vi "Compile Save Data (SubVI).vi"(0 "Dispense Mode":T5(ring), 1 "Mass Chart":T4, 2 "Relay Control":T2, 3 "Dispense Setpoint (%)":dbl=2.5, 4 "Values":T6 {"Drain Time (s)" format="%.2f"; "Drain Rate (g/sec)" format="%.2f"; "Spray Mass Loss (g)" format="%.2f"; "Time Elapsed (s)" format="%.2f"; "Time Target (s)" format="%.2f"; "Dynamic Setpoint (g)" format="%.2f"; "Static Setpoint (g)" format="%.2f"; "Grams to Setpoint" format="%.2f"; "Adjusted Mass (g)" format="%.2f"; "Dispense Rate (g/sec)" format="%.2f"; "Fill Mass (g)" format="%.2f"; "Fill Rate (g/sec)" format="%.2f"}, 5 "Settings":T1={"ON Settings"={"Enable Dynamic Setpoint?"=TRUE, "Enable Dynamic Dispense Time?"=TRUE, "Enable Drain Rate Functions"=TRUE, "Dispense Sample Time (s)"=0.1, "Mass Average Samples"=20, "ON Timeout (sec)"=300.0, "1st Setpoint (% of Target)"=90.0, "2nd Setpoint (% of Target)"=95.0, "3rd Setpoint (% of Target)"=100.0, "Measure Dispense Delay (sec)"=10.0, "Minimum Spray Time (s)"=2.0, "Pump Reverse Time (s)"=10.0}, "OFF Settings"={"Drain Sample Time (s)"=0.1, "Drain Rate Ave Size"=100, "Drain Rate Limits (± g/sec)"=100.0, "Level Slope Range (± g/sec)"=0.05, "OFF Timeout (sec)"=300.0, "Near SP Slope Level (± g/sec)"=0.005, "Near Setpoint Threshold (%)"=99.0}, "Overshoot Settings"={"Time Limit (s)"=30.0, "Container MAX (g)"=1500.0, "Max FILL Slope (+/- g/sec)"=100.0, "% Overshot to Enable (>)"=3.0}, "FILL Timeout (s)"=300.0, "Full \nSettle Time (s)"=30.0, "Pre-Hydrate \nSpray Time (s)"=0.0, "Pre-Hydrate \nWait Time (s)"=10.0, "m Value "=1.0, "b Value"=0.0, "Enable Overshoot Adjust?"=FALSE} {"ON Settings"."Pump Reverse Time (s)" min=0.0 max=60.0; "OFF Settings"."Near SP Slope Level (± g/sec)" format="%.3g"; "OFF Settings"."Level Slope Range (± g/sec)" format="%.3g"}, 7 "Hydration (g)":dbl, 9 "Product Mass (g)":dbl, 11 "Product Values":T3) -> (14 "Data Array Output":string[](array[string]), 15 "Column Header Text Array":string[](array[string])=["Grams (SCB)", "Fill Target", "Dispense Target", "Relay (All)", "Relay1 (Spray)", "Relay2 (Fill)", "Relay3 (Drain)", "Relay4", "Relay5", "Relay6", "Relay7", "Dispense Mode", "Dispense Setpoint (%)", "Spray Timeout (s)", "Wait Timeout (s)", "Adjusted Mass (grams)", "Time Target (s)", "Dispense Rate (g/sec)", "Dynamic Setpoint (g)", "Measure Dispense Delay (s)", "Fill Mass (grams)", "Fill Rate (g/sec)", "Time Elapsed (s)", "Spray Mass Loss (g)"])   [LabVIEW 2011]
panel:
  # "ONLY ADJUST\nBOLD VALUES!"
  # "Corrected Mass = SDC Mass * m + b"
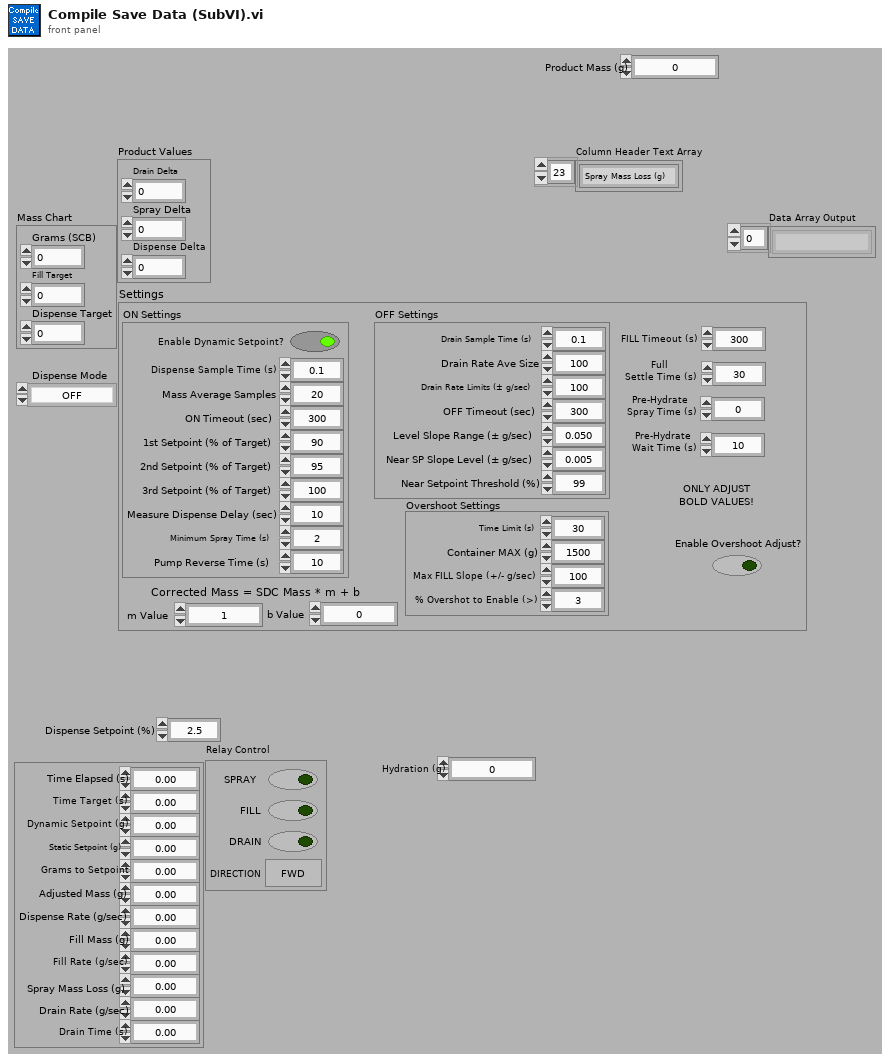
[diagram p1: front panel]
types:
  T1 = cluster{"ON Settings":cluster{"Enable Dynamic Setpoint?":bool, "Enable Dynamic Dispense Time?":bool, "Enable Drain Rate Functions":bool, "Dispense Sample Time (s)":dbl, "Mass Average Samples":i32, "ON Timeout (sec)":dbl, "1st Setpoint (% of Target)":dbl, "2nd Setpoint (% of Target)":dbl, "3rd Setpoint (% of Target)":dbl, "Measure Dispense Delay (sec)":dbl, "Minimum Spray Time (s)":dbl, "Pump Reverse Time (s)":dbl}, "OFF Settings":cluster{"Drain Sample Time (s)":dbl, "Drain Rate Ave Size":i32, "Drain Rate Limits (± g/sec)":dbl, "Level Slope Range (± g/sec)":dbl, "OFF Timeout (sec)":dbl, "Near SP Slope Level (± g/sec)":dbl, "Near Setpoint Threshold (%)":dbl}, "Overshoot Settings":cluster{"Time Limit (s)":dbl, "Container MAX (g)":dbl, "Max FILL Slope (+/- g/sec)":dbl, "% Overshot to Enable (>)":dbl}, "FILL Timeout (s)":dbl, "Full \nSettle Time (s)":dbl, "Pre-Hydrate \nSpray Time (s)":dbl, "Pre-Hydrate \nWait Time (s)":dbl, "m Value ":dbl, "b Value":dbl, "Enable Overshoot Adjust?":bool}
  T2 = cluster{"FILL":bool, "SPRAY":bool, "DIRECTION":bool, "DRAIN":bool}
  T3 = cluster{"Drain Delta":dbl, "Spray Delta":dbl, "Dispense Delta":dbl}
  T4 = cluster{"Grams (SCB)":dbl, "Fill Target":dbl, "Dispense Target":dbl}
  T5 = enum16{"OFF", "INITIAL", "FILL", "DISPENSE", "ADJUST"}
  T6 = cluster{"Time Elapsed (s)":dbl, "Time Target (s)":dbl, "Dynamic Setpoint (g)":dbl, "Static Setpoint (g)":dbl, "Grams to Setpoint":dbl, "Adjusted Mass (g)":dbl, "Dispense Rate (g/sec)":dbl, "Fill Mass (g)":dbl, "Fill Rate (g/sec)":dbl, "Spray Mass Loss (g)":dbl, "Drain Rate (g/sec)":dbl, "Drain Time (s)":dbl}
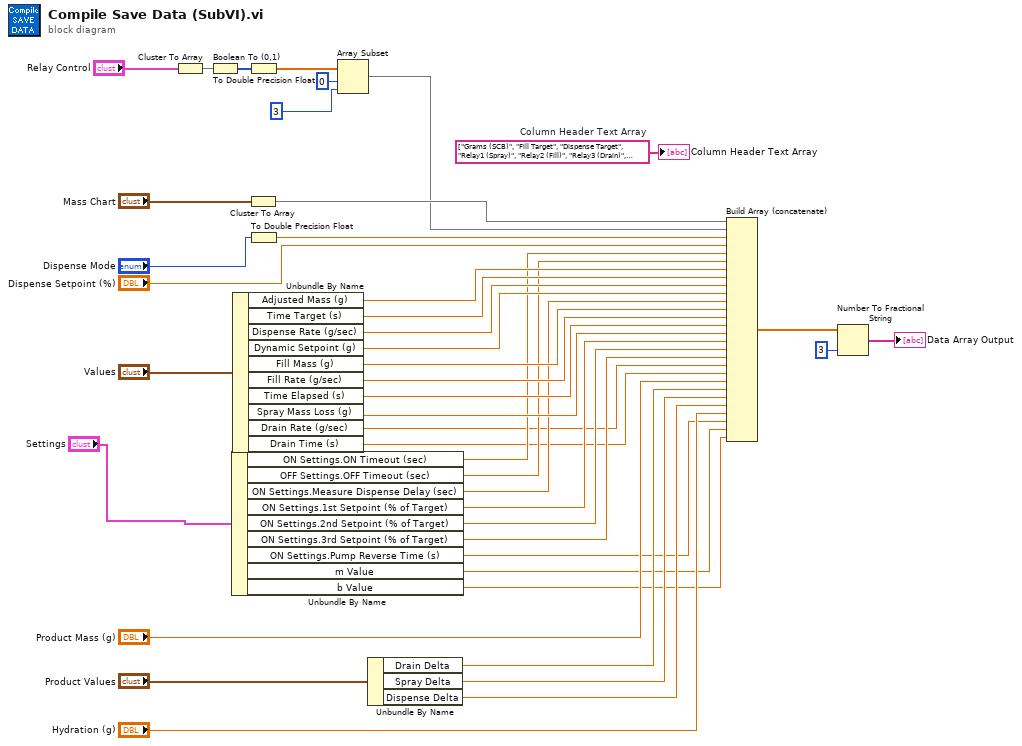
[diagram p0: block diagram]
diagram:
  w24 = string[] ["Grams (SCB)", "Fill Target", "Dispense Target", "Relay1 (Spray)", "Relay2 (Fill)", "Relay3 (Drain)", "Dispense Mode", "Dispense Setpoint (%)", "Spray Timeout (s)", "Wait Timeout (s)", "Adjusted Mass (grams)", "Time Target (s)", "Dispense Rate (g/sec)", "Dynamic Setpoint (g)", "Measure Dispense Delay (s)", "Fill Mass (grams)", "Fill Rate (g/sec)", "Time Elapsed (s)", "Spray Mass Loss (g)", "SP 1 (%)", "SP2 (%)", "SP3 (%)", "Drain Rate (g/sec)", "Drain Time (s)", "Product Mass (g)", "Drain Delta (g)", "Spray Delta (g)", "Dispense Delta (g)", "Hydration (g)", "Reverse Time (sec)", "Correction m Value", "Correction b Value"]  # Column Header Text Array
  n1 = Cluster To Array(cluster="Relay Control") -> (array=w25:bool[])
  n2 = Boolean To (0,1)(Boolean=w25) -> (0, 1=w26:i16[])
  n3 = Unbundle By Name("Settings") -> ("ON Settings.ON Timeout (sec)"=w29:dbl, "OFF Settings.OFF Timeout (sec)"=w30:dbl, "ON Settings.Measure Dispense Delay (sec)"=w31:dbl, "ON Settings.1st Setpoint (% of Target)"=w23:dbl, "ON Settings.2nd Setpoint (% of Target)"=w22:dbl, "ON Settings.3rd Setpoint (% of Target)"=w21:dbl, "ON Settings.Pump Reverse Time (s)"=w4:dbl, "m Value"=w3:dbl, "b Value"=w2:dbl)
  n4 = Unbundle By Name("Values") -> ("Adjusted Mass (g)"=w32:dbl, "Time Target (s)"=w33:dbl, "Dispense Rate (g/sec)"=w34:dbl, "Dynamic Setpoint (g)"=w35:dbl, "Fill Mass (g)"=w36:dbl, "Fill Rate (g/sec)"=w37:dbl, "Time Elapsed (s)"=w38:dbl, "Spray Mass Loss (g)"=w39:dbl, "Drain Rate (g/sec)"=w20:dbl, "Drain Time (s)"=w19:dbl)
  n5 = Cluster To Array(cluster="Mass Chart") -> (array=w27:dbl[])
  n6 = To Double Precision Float(number=w26) -> (double precision float=w18:dbl[])
  n7 = To Double Precision Float(number="Dispense Mode") -> (double precision float=w28:dbl)
  n8 = Array Subset(array=w18, index=0, length=3 ("index")) -> (w5:dbl[])
  n9 = Unbundle By Name("Product Values") -> ("Drain Delta"=w14:dbl, "Spray Delta"=w13:dbl, "Dispense Delta"=w12:dbl)
  n10 = Build Array (concatenate)(w27, w5, w28, "Dispense Setpoint (%)", w29, w30, w32, w33, w34, w35, w31, w36, w37, w38, w39, w23, w22, w21, w20, w19, "Product Mass (g)", w14, w13, w12, "Hydration (g)", w4, w3, w2) -> (w10:dbl[])
  n11 = Number To Fractional String(number=w10, precision (6)=i16 3) -> (F-format string=→"Data Array Output":string[])  [unwired: 2 in]
  "Column Header Text Array" <- w24
